vi "UI.vi"(8 "error in (no error)":errorcluster, 11 "View in":refnum<class "View.lvclass">) -> (0 "error out":errorcluster, 3 "View out":refnum<class "View.lvclass">)   [LabVIEW 2020, in "Page2.lvlib" / "View.lvclass"]
uses:
  View.lvclass
  View.lvclass/View.ctl
  Controller/Controller.lvclass
panel:
  in  "Main Test Folder":path
  in  "Setting":u32
  out "Time (s)":u32
  # "Page 2 UI"
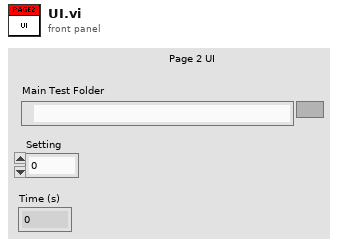
[diagram p1: front panel]
types:
  T1 = cluster{"Setting":refnum<vi>, "Time (s)":refnum<vi>, "Main Test Folder":refnum<vi>}
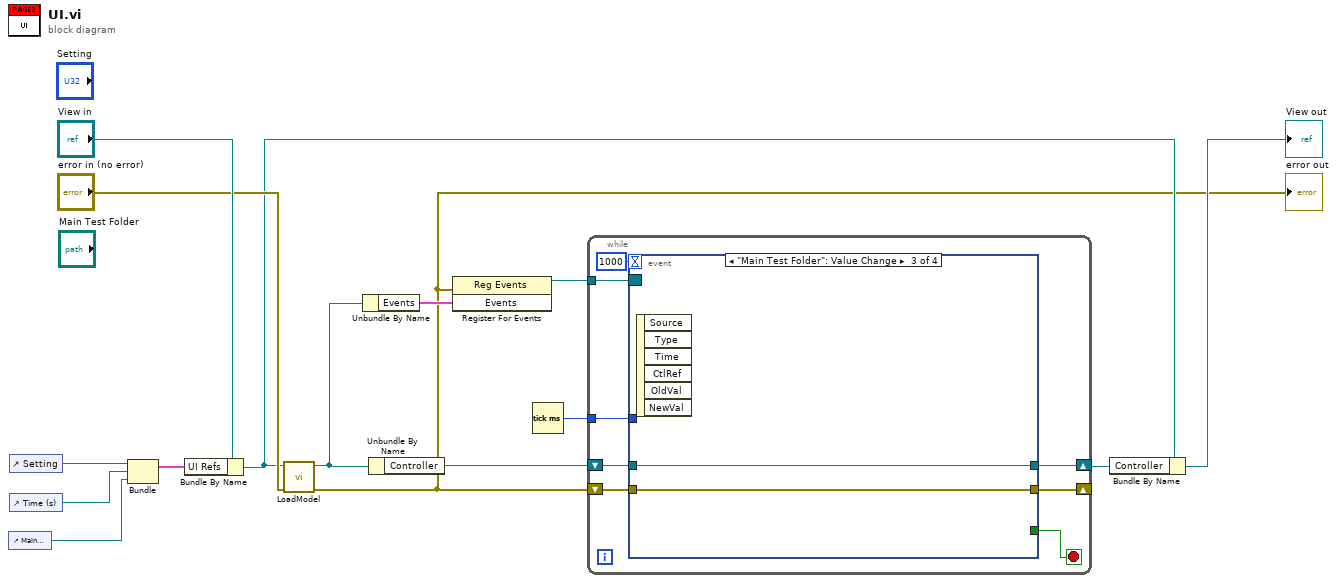
[diagram p0: block diagram]
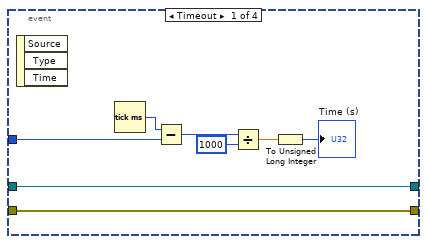
[diagram p2: hidden frame]
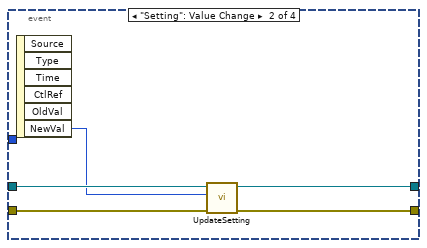
[diagram p3: hidden frame]
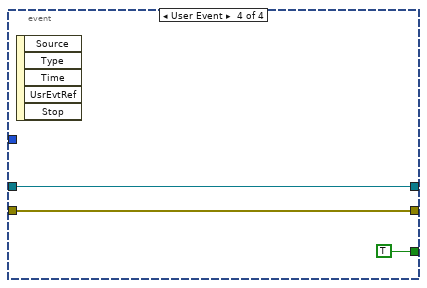
[diagram p4: hidden frame]
diagram:
  n1 = control-ref of="Main Test Folder"() -> (w8:refnum<vi>)
  n2 = control-ref of="Setting"() -> (w12:refnum<vi>)
  n3 = control-ref of="Time (s)"() -> (w11:refnum<vi>)
  n4 = Bundle("Setting"=w12, "Time (s)"=w11, "Main Test Folder"=w8) -> (w10:T1)  [unwired: 1 in]
  n5 = Bundle By Name(cluster="View in", "UI Refs"=w10) -> (w4:refnum<class "View.lvclass">)
  n6 = call "LoadModel.vi"("error in (no error)"="error in (no error)", "View in"=w4) -> ("error out"=w1:errorcluster, "View out"=w6:refnum<class "View.lvclass">)  [unwired: 8 in]
  "error out" <- w1
  n7 = Unbundle By Name(w6) -> ("Events"=w15:cluster{"Stop":refnum<user-event>})
  n8 = Unbundle By Name(w6) -> ("Controller"=w5:refnum<class "Controller.lvclass">)
  n9 = register-events(error in=w1, w15) -> (reference out=w14:refnum<event-registration>)  [unwired: 1 in, 1 out]
  n10 = Tick Count (ms)() -> (millisecond timer value=w13:u32)
  n11 = while {
    tunnel: w14 -> [w23]
    tunnel: w13 -> [w20]
    shift-right: [w18] -> w3
    shift-left: w5 -> [w19]
    shift-right: [w16] -> _
    shift-left: w1 -> [w17]
    stop <- w22 stop-if-true
    n12 = event shown="[2] \"Main Test Folder\": Value Change" {
      selector: w23 -> [_ _ _ _]
      dyn-events: _ -> [_ _ _ _]
      timeout: 1000 -> [_ _ _ _]
      tunnel: [_ _ _ TRUE] -> w22
      tunnel: w20 -> [w30 _ _ _]
      tunnel: w19 -> [w25 w36 w38 w40]
      tunnel: [w25 w35 w38 w40] -> w18
      tunnel: w17 -> [w24 w34 w37 w39]
      tunnel: [w24 w33 w37 w39] -> w16
      event Timeout {
        n13 = event-data() -> ()  [unwired: 1 in, 3 out]
        n14 = Tick Count (ms)() -> (millisecond timer value=w31:u32)
        n15 = Subtract(x=w31, y=w30) -> (x-y=w29:u32)
        n16 = Divide(x=w29, y=u32 1000) -> (x/y=w28:dbl)
        n17 = To Unsigned Long Integer(number=w28) -> (unsigned 32bit integer=→"Time (s)":u32)
      }
      event "Setting": Value Change {
        n18 = event-data() -> ("NewVal"=w32:u32)  [unwired: 1 in, 5 out]
        n19 = call "UpdateSetting.vi"("error in (no error)"=w34, "Setting"=w32, "Controller in"=w36) -> ("error out"=w33:errorcluster, "Controller out"=w35:refnum<class "Controller.lvclass">)  [unwired: 7 in]
      }
      event "Main Test Folder": Value Change {
        n20 = event-data() -> ()  [unwired: 1 in, 6 out]
      }
      event User Event {
        n21 = event-data() -> ()  [unwired: 1 in, 5 out]
      }
    }
  }
  n22 = Bundle By Name(cluster=w4, "Controller"=w3) -> (→"View out":refnum<class "View.lvclass">)
